vi "myRIO_BRig_RT_dataBlock_targetTpB__L.vi"() -> (2 "output_targetTpB__L":i32)   [LabVIEW 2014]
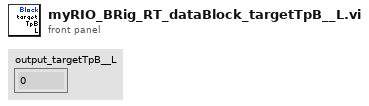
[diagram p1: front panel]
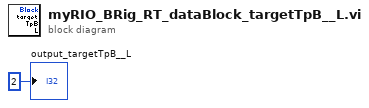
[diagram p0: block diagram]
diagram:
  "output_targetTpB__L" <- 2 ("output_iBlock")
